vi "Get Samples Per Cycle.vi"(2 "gen":refnum<class "niUSRP Tx DSP v2 FPGA.lvclass">) -> (4 "samples per cycle":u16)   [LabVIEW 2025, in "niUSRP Tx DSP v2 FPGA.lvclass"]
doc: "this VI returns the number of samples per cycle (spc) generated by this device at the DAC output."
uses:
  niUSRP Tx DSP v2 FPGA.lvclass
  niUSRP Tx DSP v2 FPGA.lvclass/niUSRP Tx DSP v2 FPGA.ctl
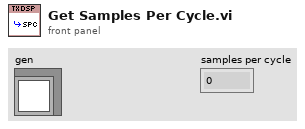
[diagram p1: front panel]
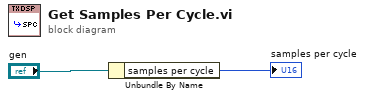
[diagram p0: block diagram]
diagram:
  n1 = Unbundle By Name("gen") -> ("samples per cycle"=→"samples per cycle":u16)
